vi "Write Headers.vi"(7 "Linked List ID":string, 8 "error in (no error)":errorcluster, 9 "Header Values":string[](array[string]), 10 "Header Names":string[](array[string]), 11 "Linked List in":refnum<class "Linked List.lvclass">) -> (0 "error out":errorcluster, 3 "Linked List out":refnum<class "Linked List.lvclass">)   [LabVIEW 2019, in "Linked Lists.lvlib" / "Linked List.lvclass"]
uses:
  <vilib>/gpm_packages/@cs/linked-list/Source/Linked List/Linked List/Linked List.lvclass
  <vilib>/gpm_packages/@cs/linked-list/Source/Linked List/Linked List Definition/Linked List Definition.lvclass
  <vilib>/gpm_packages/@cs/linked-list/Source/Linked List/Linked List/Linked List.lvclass/Linked List.ctl
  <vilib>/gpm_packages/@cs/lookup-table/Source/LookupTable/LookupTable.lvclass/LookupTable.ctl
  1d08a9d6-ec4b-4164-8abc-acf90aac6253.vi
  <vilib>/gpm_packages/@cs/lookup-table/Source/LookupTable/Read Table Reference.vi
  1d08a9d6-ec4b-4164-8abc-acf90aac6253.vi/bf5b6fc5-7452-4c1b-8065-dbe71e8cd3b6.vi
  <vilib>/gpm_packages/@cs/lookup-table/Source/LookupTable/LookupTable.lvclass
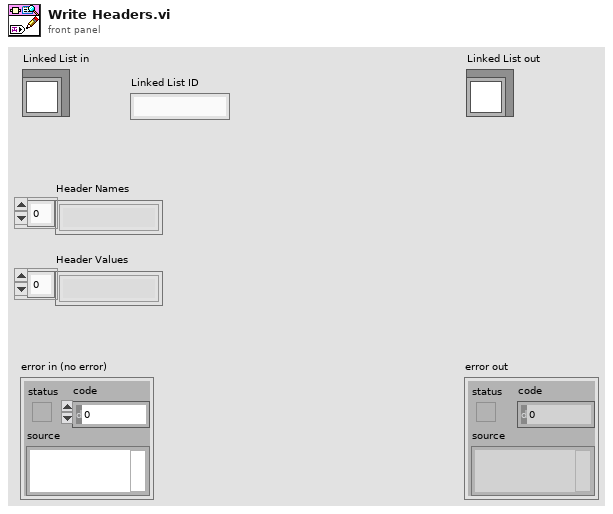
[diagram p1: front panel]
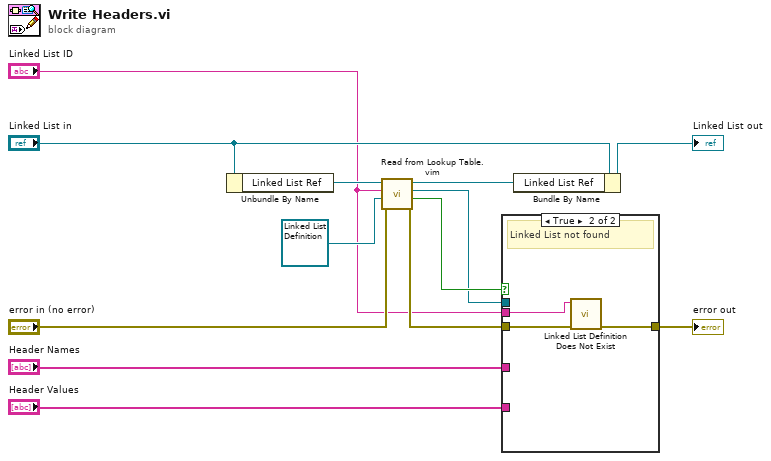
[diagram p0: block diagram]
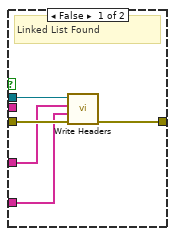
[diagram p2: hidden frame]
diagram:
  n1 = Unbundle By Name("Linked List in") -> ("Linked List Ref"=w13:refnum<data-value>)
  n2 = call "Read from Lookup Table.vim"("error in (no error)"="error in (no error)", "Type"=refnum<class "Linked List Definition.lvclass"> refnum ("Linked List.lvlib:Linked List Definition.lvclass"), "Item Name"="Linked List ID", "LookupTable Reference"=w13) -> ("error out"=w5:errorcluster, "Not Found?"=w7:bool, "Value"=w6:refnum<class "Linked List Definition.lvclass">, "LookupTable Reference Out"=w11:refnum<data-value>)  [unwired: 4 in]
  n3 = case shown="True" w7 {
    tunnel: w6 -> [w18 _]
    tunnel: w5 -> [w17 w21]
    tunnel: [w14 w20] -> w4
    tunnel: "Header Names" -> [w16 _]
    tunnel: "Header Values" -> [w15 _]
    tunnel: "Linked List ID" -> [_ w19]
    frame False {
      # "Linked List Found"
      n4 = call <vilib>:"Write Headers.vi"("error in (no error)"=w17, "Header Values"=w15, "Header Names"=w16, "Linked List Definition in"=w18) -> ("error out"=w14:errorcluster)  [unwired: 6 in, 1 out]
    }
    frame True {
      # "Linked List not found"
      n5 = call <vilib>:"Linked List Definition Does Not Exist.vi"("Error In"=w21, "Unique ID"=w19) -> ("Error Out"=w20:errorcluster)  [unwired: 9 in]
    }
  }
  "error out" <- w4
  n6 = Bundle By Name(cluster="Linked List in", "Linked List Ref"=w11) -> (→"Linked List out":refnum<class "Linked List.lvclass">)
